vi "Front Panel DataSocket - Writer.vi"() -> ()   [LabVIEW 2023]
doc: "Uses DataSocket to publish data to the DataSocket Server on the local machine. The waveform graph on the front panel is configured to publish its data to a DataSocket Server on the local computer. When the VI runs, the control connects to the DataSocket Server and sends data to it.\n\nTo set up the DataSocket connection of the waveform graph, right-click the waveform graph and select Properties and go to the Data Binding tab."
panel:
  in  "Stop":bool
  out "Data Written":dbl[](graph)
  # "Overview: Demonstrates the use of DataSocket front panel binding to write data to the DataSocket server.\nRequirements: Windows\nInstructions:\n1. Run the DataSocket server by navigating the Windows start menu to National Instruments > DataSocket > DataSocket Server.\n2. Run the VI.\n3. Open Front Panel DataSocket - Reader.vi and follow the instructions on its front panel.\n4. Click Stop to stop the VI."
  # "Right-click the graph and choose Properties, then select the Data Binding tab, to configure the graph to publish its data to the DataSocket server. This graph is configured to publish its data to the following URL:\n\ndstp://localhost/fpwave\n\nNote that the connection status LED in the upper-right corner of the graph will turn green when the VI runs and a DataSocket connection is established."
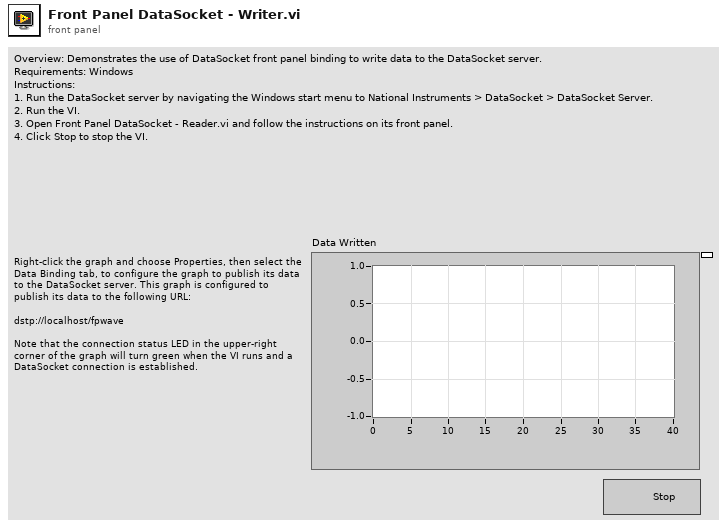
[diagram p1: front panel]
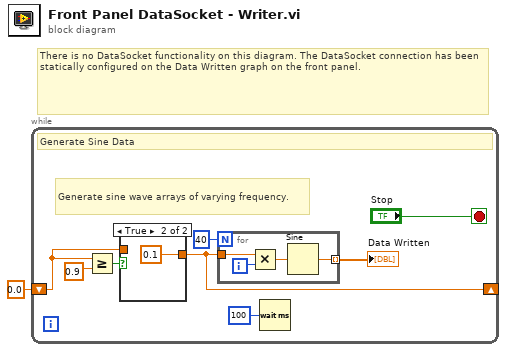
[diagram p0: block diagram]
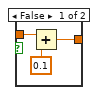
[diagram p2: hidden frame]
diagram:
  # "There is no DataSocket functionality on this diagram. The DataSocket connection has been statically configured on the Data Written graph on the front panel."
  n1 = while {
    shift-left: 0.0 -> [w8]
    shift-right: [w7] -> _
    stop <- "Stop" stop-if-true
    # "Generate sine wave arrays of varying frequency."
    # "Generate Sine Data"
    n2 = Greater Or Equal?(x=w8, y=0.9) -> (x >= y?=w4:bool)
    n3 = case shown="True" w4 {
      tunnel: [w15 0.1] -> w7
      tunnel: w8 -> [w16 _]
      frame False {
        n4 = Add(x=w16, y=0.1) -> (x+y=w15:dbl)
      }
      frame True {
      }
    }
    n5 = for {
      N: 40 -> [_]
      tunnel: w7 -> [w13]
      tunnel: [w10] -> w2 mode=indexing
      i -> [w12]
      n6 = Multiply(x=w13, y=w12) -> (x*y=w11:dbl)
      n7 = Sine(x=w11) -> (sin(x)=w10:dbl)
    }
    "Data Written" <- w2
    n8 = Wait (ms)(milliseconds to wait=u32 100) -> ()  [unwired: 1 out]
  }
